vi "Update Static Overlays.vi"(8 "error in (no error)":errorcluster, 10 "Static Overlay.lvclass":refnum<class "Static Overlay.lvclass">, 11 "HIJ Vision Application in":refnum<class "HIJ Vision Application.lvclass">) -> (0 "error out":errorcluster, 3 "HIJ Vision Application out":refnum<class "HIJ Vision Application.lvclass">)   [LabVIEW 2020, in "HIJ Vision Application.lvlib" / "HIJ Vision Application.lvclass"]
uses:
  HIJ Vision Application.lvclass
  Analyze/Results and Overlays/Static Overlay/Static Overlay.lvclass
  HIJ Vision Application.lvclass/HIJ Vision Application.ctl
  Display Actors/HIJ Vision Display/HIJ Vision Display Messages/Update Static Overlay Msg/Update Static Overlay Msg.lvclass/Update Static Overlay Msg.ctl
  <vilib>/ActorFramework/Message Enqueuer/Message Enqueuer.lvclass/Message Enqueuer.ctl
  <vilib>/ActorFramework/Message Enqueuer/Enqueue.vi
  Display Actors/HIJ Vision Display/HIJ Vision Display Messages/Update Static Overlay Msg/Update Static Overlay Msg.lvclass
  C:/Program Files (x86)/National Instruments/LabVIEW 2020/vi.lib/ActorFramework/Message/Message.lvclass
  <vilib>/ActorFramework/Message Priority Queue/Priority Enqueue.vi
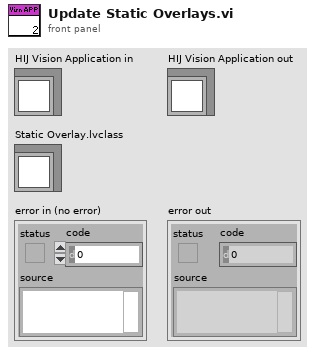
[diagram p1: front panel]
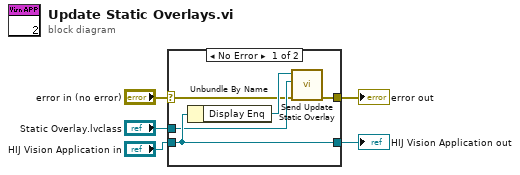
[diagram p0: block diagram]
diagram:
  n1 = case shown="No Error" "error in (no error)" {
    selector: "error in (no error)" -> [w7 w12]
    tunnel: [w6 w12] -> w4
    tunnel: [w10 w11] -> w2
    tunnel: "HIJ Vision Application in" -> [w10 w11]
    tunnel: "Static Overlay.lvclass" -> [w8 _]
    frame No Error {
      n2 = Unbundle By Name(w10) -> ("Display Enq"=w9:refnum<class "Message Enqueuer.lvclass">)
      n3 = call "Send Update Static Overlay.vi"("error in (no error)"=w7, "Static Overlay"=w8, "Message Enqueuer"=w9) -> ("error out"=w6:errorcluster)  [unwired: 7 in, 1 out]
    }
    frame Error {
    }
  }
  "error out" <- w4
  "HIJ Vision Application out" <- w2
